vi "Digit to Color Converter.vi"(4 "D select":T1 caption="Digit select") -> (1 "D Color":u32(colorbox) caption="Digit Color")   [LabVIEW 2018, in "Enum to Color Converters.lvlib"]
doc: "Converts the selected Digit Enum value into the corresponding color for the resistor band."
uses:
  Enum to Color Converters.lvlib
  Digit--enum.ctl
  Resistor Band Colors/Resistor Band Colors.lvlib
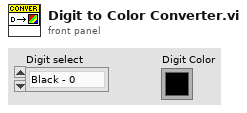
[diagram p1: front panel]
types:
  T1 = typedef "digit--enum.ctl" = enum16{"Black - 0", "Brown - 1", "Red - 2", "Orange - 3", "Yellow - 4", "Green - 5", "Blue - 6", "Violet - 7", "Grey - 8", "White - 9"}
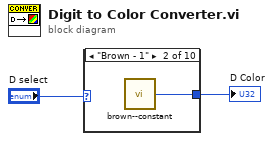
[diagram p0: block diagram]
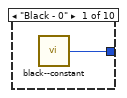
[diagram p2: hidden frame]
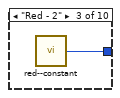
[diagram p3: hidden frame]
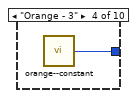
[diagram p4: hidden frame]
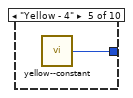
[diagram p5: hidden frame]
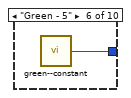
[diagram p6: hidden frame]
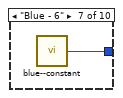
[diagram p7: hidden frame]
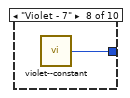
[diagram p8: hidden frame]
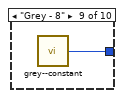
[diagram p9: hidden frame]
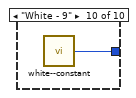
[diagram p10: hidden frame]
diagram:
  n1 = case shown="\"Brown - 1\"" "D select" {
    tunnel: [w3 w4 w5 w6 w7 w8 w9 w10 w11 w12] -> w1
    frame "Black - 0" {
      n2 = call "black--constant.vi"() -> ("Black"=w3:u32)  [unwired: 5 in]
    }
    frame "Brown - 1" {
      n3 = call "brown--constant.vi"() -> ("Brown"=w4:u32)  [unwired: 5 in]
    }
    frame "Red - 2" {
      n4 = call "red--constant.vi"() -> ("Red"=w5:u32)  [unwired: 5 in]
    }
    frame "Orange - 3" {
      n5 = call "orange--constant.vi"() -> ("Orange"=w6:u32)  [unwired: 5 in]
    }
    frame "Yellow - 4" {
      n6 = call "yellow--constant.vi"() -> ("Yellow"=w7:u32)  [unwired: 5 in]
    }
    frame "Green - 5" {
      n7 = call "green--constant.vi"() -> ("Green"=w8:u32)  [unwired: 5 in]
    }
    frame "Blue - 6" {
      n8 = call "blue--constant.vi"() -> ("Blue"=w9:u32)  [unwired: 5 in]
    }
    frame "Violet - 7" {
      n9 = call "violet--constant.vi"() -> ("Violet"=w10:u32)  [unwired: 5 in]
    }
    frame "Grey - 8" {
      n10 = call "grey--constant.vi"() -> ("Gray"=w11:u32)  [unwired: 5 in]
    }
    frame "White - 9" {
      n11 = call "white--constant.vi"() -> ("White"=w12:u32)  [unwired: 5 in]
    }
  }
  "D Color" <- w1
